vi "Disable.vi"(11 "Ctl Refnum":refnum<vi>) -> (3 "Ctl Refnum Out":refnum<vi>)   [LabVIEW 2024]
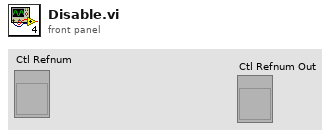
[diagram p1: front panel]
types:
  T1 = enum8{"Enabled", "Disabled", "Disabled and Grayed Out"}
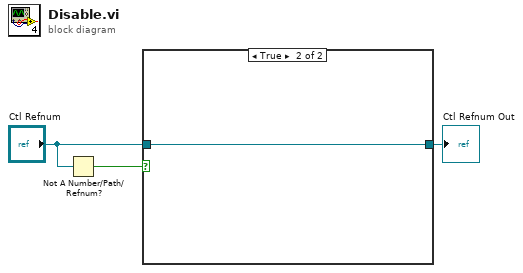
[diagram p0: block diagram]
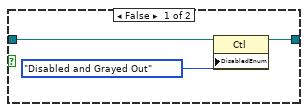
[diagram p2: hidden frame]
diagram:
  n1 = Not A Number/Path/Refnum?(number/path/refnum="Ctl Refnum") -> (NaN/Path/Refnum?=w2:bool)
  n2 = case shown="True" w2 {
    tunnel: "Ctl Refnum" -> [w5 w7]
    tunnel: [w4 w7] -> w1
    frame False {
      n3 = property class="Ctl"(reference=w5, "DisabledEnum"=T1."Disabled and Grayed Out" ("Disabled")) -> (reference out=w4:refnum<vi>)  [unwired: 1 in, 1 out]
    }
    frame True {
    }
  }
  "Ctl Refnum Out" <- w1
